vi "grabSetup_action.vi"(0 "HGF_ImaqFg":refnum<class "HGF_ImaqFg.lvclass">, 5 "error in (no error)":errorcluster, 6 "Region of Interest":i32[](array[numeric]), 7 "Step x":i32=-1, 8 "Channel":i32=-1, 9 "Step y":i32=-1) -> (14 "dup HGF_ImaqFg":refnum<class "HGF_ImaqFg.lvclass">, 19 "error out":errorcluster)   [LabVIEW 2014, in "HGF_IMAQ.lvlib" / "HGF_ImaqFg.lvclass"]
doc: "Starts a grab acquisition. This VI performs a continuous acquisition that provides access to the most recently acquired image.\n\nParameter are used for framegrabber, only, and can be ignored for IMAQdx and IMAQ for USB."
uses:
  HGF_ImaqFg.lvclass
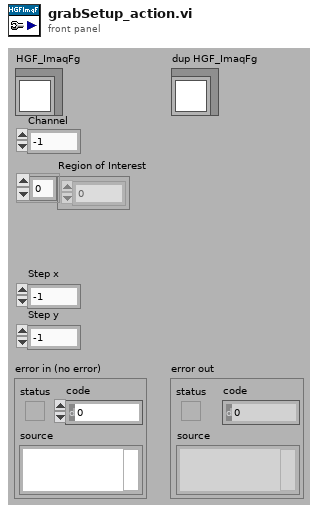
[diagram p1: front panel]
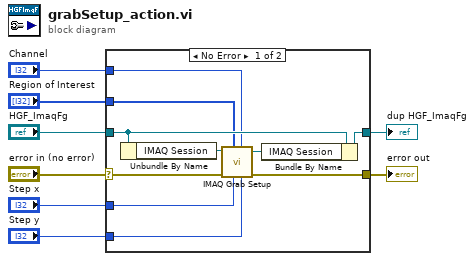
[diagram p0: block diagram]
diagram:
  n1 = case shown="No Error" "error in (no error)" {
    selector: "error in (no error)" -> [w9 w19]
    tunnel: "HGF_ImaqFg" -> [w17 w20]
    tunnel: [w15 w20] -> w7
    tunnel: [w14 w19] -> w6
    tunnel: "Region of Interest" -> [w13 _]
    tunnel: "Channel" -> [w12 _]
    tunnel: "Step x" -> [w11 _]
    tunnel: "Step y" -> [w10 _]
    frame No Error {
      n2 = Unbundle By Name(w17) -> ("IMAQ Session"=w18:refnum<k11>)
      n3 = call <vilib>:"IMAQ Grab Setup.vi"("Step y"=w10, "Channel"=w12, "Step x"=w11, "Region of Interest"=w13, "error in (no error)"=w9, "IMAQ Session In"=w18) -> ("error out"=w14:errorcluster, "IMAQ Session Out"=w16:refnum<k11>)  [unwired: 4 out]
      n4 = Bundle By Name(cluster=w17, "IMAQ Session"=w16) -> (w15:refnum<class "HGF_ImaqFg.lvclass">)
    }
    frame Error {
    }
  }
  "error out" <- w6
  "dup HGF_ImaqFg" <- w7
